vi "Generic LV App Config Save-Retrieve.vi"(8 "error in":errorcluster, 11 "Save/Retrieve":string(combo)="Retrieve") -> (0 "error out":errorcluster, 1 "Path to conf file":path, 2 "Calling VI's Controls":string[](array[string]), 3 "Refs to Calling VI's controls":refnum<vi>[](array[refnum]), 4 "Controls updated":string[](array[string]))   [LabVIEW 2023]
uses:
  <vilib>/Utility/sysdir.llb/System Directory Type.ctl
  <vilib>/Utility/error.llb/Trim Whitespace One-Sided.vi
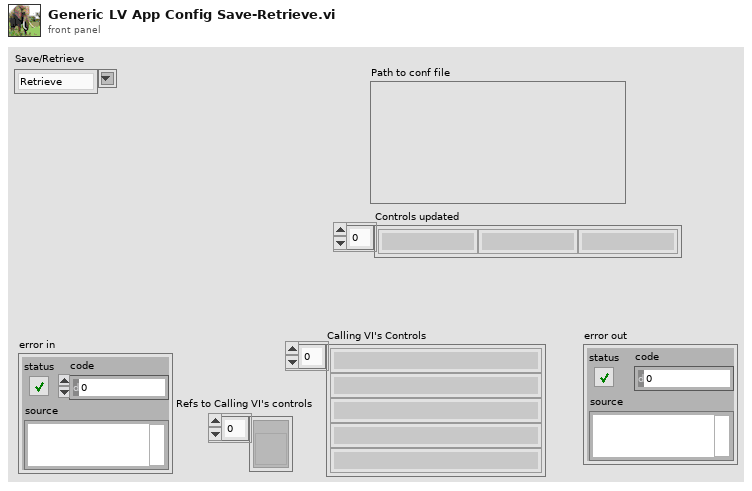
[diagram p1: front panel]
types:
  T1 = enum16{"open", "replace", "create", "open or create", "replace or create", "replace or create with confirmation"}
  T2 = typedef "System Directory Type.ctl" = i32
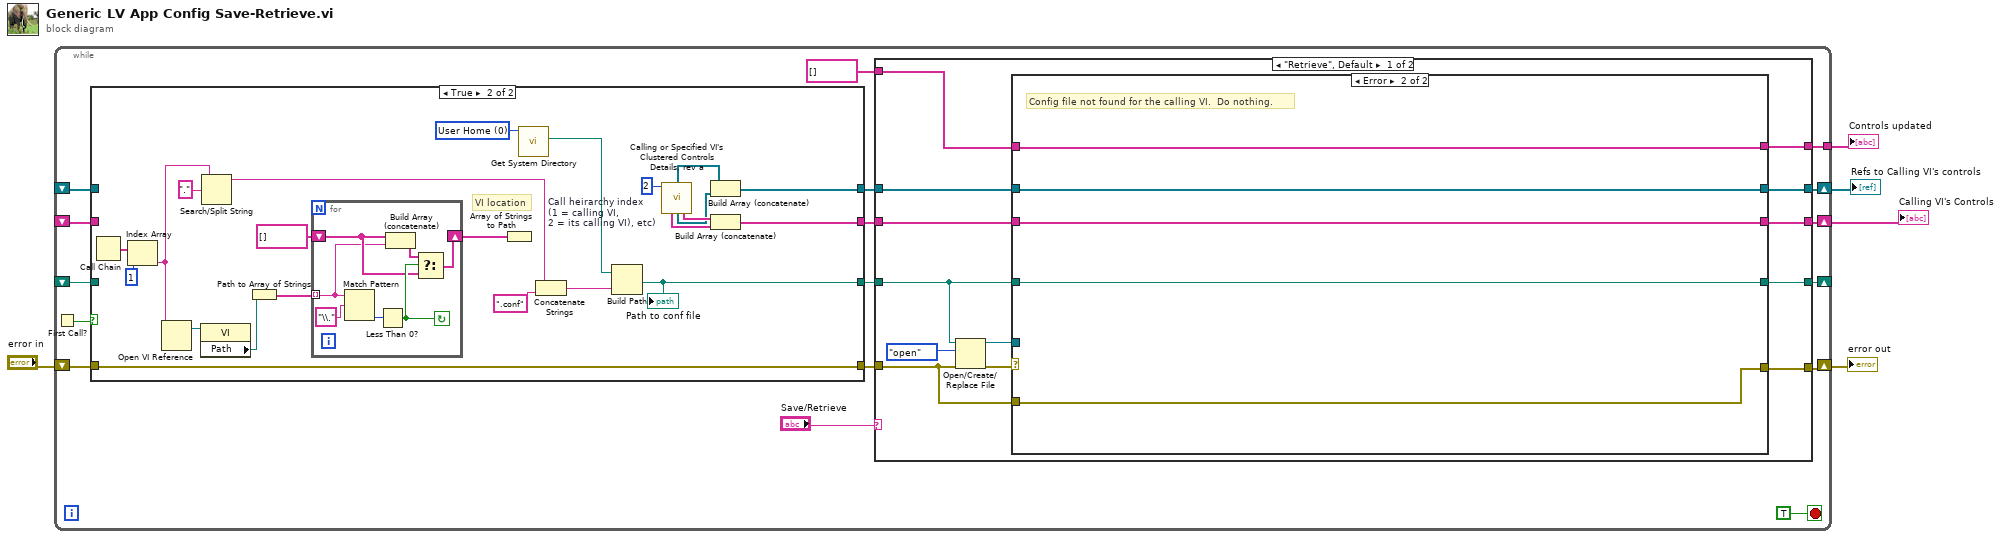
[diagram p0: block diagram]
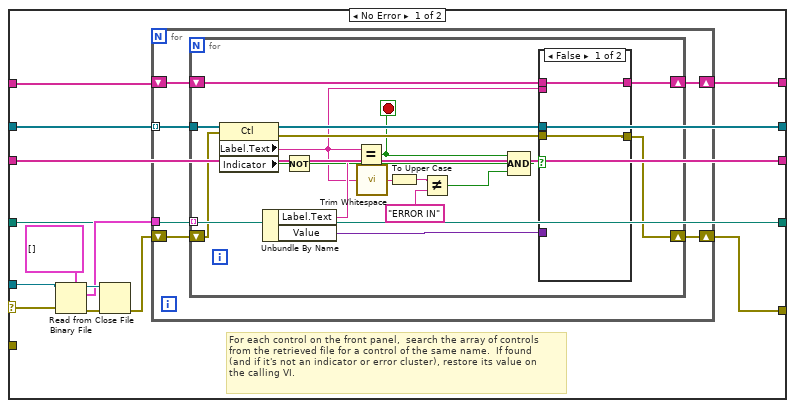
[diagram p3: hidden frame]
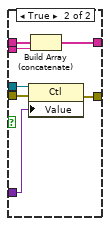
[diagram p4: hidden frame]
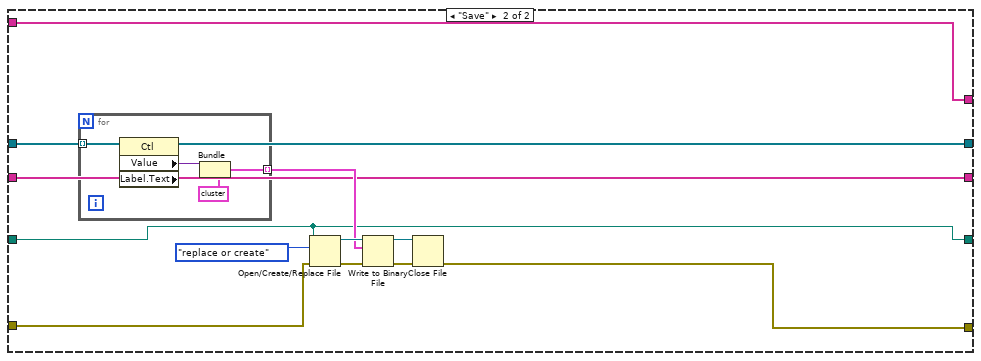
[diagram p5: hidden frame]
diagram:
  n1 = while {
    shift-right: [w15] -> w4
    shift-left: "error in" -> [w18]
    shift-right: [w16] -> w3
    shift-left: _ -> [w12]
    shift-right: [w13] -> w2
    shift-left: _ -> [w11]
    shift-right: [w10] -> _
    shift-left: _ -> [w9]
    tunnel: [w7] -> w1
    stop <- TRUE stop-if-true
    n2 = First Call?() -> (First Call?: T/F=w17:bool)
    n3 = case shown="True" w17 {
      tunnel: [w26 w43] -> w22
      tunnel: [w24 w41] -> w21
      tunnel: [w23 w40] -> w20
      tunnel: w18 -> [w23 w40]
      tunnel: [w25 w39] -> w14
      tunnel: w12 -> [w26 _]
      tunnel: w11 -> [w25 _]
      tunnel: w9 -> [w24 _]
      frame False {
      }
      frame True {
        w28 = T2 0 items=["User Home"=0, "User Desktop"=1, "User Documents"=2, "User Application Data"=3, "User Preferences"=4, "User Temporary"=5, "Public Documents"=6, "Public Application Data"=7, "Public Preferences"=8, "Public Cache"=13, "System Core Libraries"=9, "System Installed Libraries"=10, "Application Files"=11, "Boot Volume Root"=12] ("system directory type")
        w38 = 2  # Call heirarchy index (1 = calling VI,  2 = its calling VI), etc)
        # "VI location"
        n4 = Call Chain() -> (call chain=w49:string[])
        n5 = Index Array(array=w49, index=1) -> (element=w34:string)
        n6 = Open VI Reference(vi path=w34) -> (vi reference=w37:refnum<vi>)  [unwired: 5 in, 1 out]
        n7 = property class="VI"(reference=w37) -> ("Path"=w32:path)  [unwired: 1 in, 2 out]
        n8 = Search/Split String(string=w34, search string/char (-)=".") -> (substring before match=w33:string)  [unwired: 1 in, 2 out]
        n9 = Path to Array of Strings(0:w32) -> (2:w30:string[])  [unwired: 1 out]
        n10 = for {
          tunnel: w30 -> [w50] mode=indexing
          shift-right: [w52] -> w29
          shift-left: string[] [] -> [w51]
          stop <- w54 continue-if-true
          n11 = Match Pattern(string=w50, regular expression="\\.") -> (offset past match=w55:i32)  [unwired: 1 in, 3 out]
          n12 = Less Than 0?(x=w55) -> (x < 0?=w54:bool)
          n13 = Build Array (concatenate)(w51, w50) -> (w53:string[])
          n14 = Select(t=w53, s=w54, f=w51) -> (s? t:f=w52:string[])
        }
        n15 = Array of Strings to Path(0:w29) -> ()  [unwired: 1 in, 1 out]
        n16 = call <vilib>:"Get System Directory.vi"("system directory type"=w28) -> ("system directory"=w27:path)  [unwired: 10 in]
        n17 = Concatenate Strings(w33, ".conf" ("string")) -> (w36:string)
        n18 = Build Path(base path=w27, name or relative path=w36) -> (appended path=w41:path)
        "Path to conf file" <- w41
        n19 = call "Calling or Specified VI's Clustered Controls Details, rev a.vi"("Call heirarchy index\n(1 = calling VI, \n2 = its calling VI), etc)"=w38) -> ("Refs to controls on panel"=w44:refnum<vi>[], "Controls directly on tab panes"=w47:string[], "Refs to controls directly on tab panes"=w45:refnum<vi>[], "Controls on panel"=w46:string[])  [unwired: 5 in, 6 out]
        n20 = Build Array (concatenate)(w44, w45) -> (w43:refnum<vi>[])
        n21 = Build Array (concatenate)(w46, w47) -> (w39:string[])
      }
    }
    n22 = case shown="\"Retrieve\", Default" "Save/Retrieve" {
      tunnel: w22 -> [w66 w124]
      tunnel: w21 -> [w60 w123]
      tunnel: w20 -> [w67 w127]
      tunnel: [w64 w124] -> w16
      tunnel: [w63 w126] -> w15
      tunnel: w14 -> [w62 w125]
      tunnel: [w61 w125] -> w13
      tunnel: [w59 w123] -> w10
      tunnel: [w58 w122] -> w7
      tunnel: string[] [] -> [w57 w122]
      frame "Retrieve", Default {
        n23 = Open/Create/Replace File(file path (use dialog)=w60, error in=w67, operation (0:open)=T1."open") -> (refnum out=w65:refnum<file>, error out=w68:errorcluster)  [unwired: 3 in, 1 out]
        n24 = case shown="Error" w68 {
          selector: w68 -> [w82 _]
          tunnel: w67 -> [_ w121]
          tunnel: [w76 w121] -> w63
          tunnel: w66 -> [w74 w120]
          tunnel: w65 -> [w81 _]
          tunnel: [w74 w120] -> w64
          tunnel: w62 -> [w73 w119]
          tunnel: [w73 w119] -> w61
          tunnel: [w72 w118] -> w59
          tunnel: w60 -> [w72 w118]
          tunnel: [w71 w117] -> w58
          tunnel: w57 -> [w70 w117]
          frame No Error {
            # "For each control on the front panel,  search the array of controls\nfrom the retrieved file for a control of the same name.  If found\n(and if it's not an indicator or error cluster), restore its value on \nthe calling VI."
            n25 = Read from Binary File(5:cluster{"Value":variant, "Label.Text":string}[] [], 8:w82, 11:w81) -> (0:w80:errorcluster, 2:w75:cluster{"Value":variant, "Label.Text":string}[], 3:w79:refnum<file>)  [unwired: 3 in, 1 out]
            n26 = Close File(refnum=w79, error in=w80) -> (error out=w77:errorcluster)  [unwired: 1 out]
            n27 = for {
              tunnel: w74 -> [w88] mode=indexing
              tunnel: w75 -> [w87]
              shift-right: [w85] -> w76
              shift-left: w77 -> [w86]
              shift-right: [w84] -> w71
              shift-left: w70 -> [w83]
              n28 = for {
                tunnel: w88 -> [w107]
                tunnel: w87 -> [w92] mode=indexing
                shift-right: [w101] -> w85
                shift-left: w86 -> [w103]
                shift-right: [w90] -> w84
                shift-left: w83 -> [w89]
                stop <- w99 stop-if-true
                n29 = property class="Ctl"(reference=w107, error in=w103) -> (reference out=w105:refnum<vi>, error out=w102:errorcluster, "Label.Text"=w91:string, "Indicator"=w100:bool)
                n30 = Unbundle By Name(w92) -> ("Label.Text"=w106:string, "Value"=w104:variant)
                n31 = Not(x=w100) -> (.not. x?=w98:bool)
                n32 = Equal?(x=w91, y=w106) -> (x = y?=w99:bool)
                n33 = call <vilib>:"Trim Whitespace.vi"("string"=w91) -> ("trimmed string"=w96:string)  [unwired: 1 in]
                n34 = To Upper Case(1:w96) -> (0:w95:string)
                n35 = Not Equal?(x=w95, y="ERROR IN") -> (x != y?=w93:bool)
                n36 = Compound Arithmetic op=AND(w99, w98, w93) -> (w97:bool)
                n37 = case shown="False" w97 {
                  tunnel: w105 -> [_ w116]
                  tunnel: w104 -> [_ w115]
                  tunnel: w102 -> [w109 w114]
                  tunnel: [w109 w113] -> w101
                  tunnel: w91 -> [_ w112]
                  tunnel: [w108 w111] -> w90
                  tunnel: w89 -> [w108 w110]
                  frame False {
                  }
                  frame True {
                    n38 = property class="Ctl"(reference=w116, error in=w114, "Value"=w115) -> (error out=w113:errorcluster)  [unwired: 1 out]
                    n39 = Build Array (concatenate)(w110, w112) -> (w111:string[])
                  }
                }
              }
            }
          }
          frame Error {
            # "Config file not found for the calling VI.  Do nothing."
          }
        }
      }
      frame "Save" {
        n40 = for {
          tunnel: w124 -> [w138] mode=indexing
          tunnel: [w134] -> w130 mode=indexing
          n41 = property class="Ctl"(reference=w138) -> ("Value"=w137:variant, "Label.Text"=w136:string)  [unwired: 1 in, 2 out]
          n42 = Bundle(cluster=cluster{"Value":variant, "Label.Text":string} {"Value"=variant, "Label.Text"=""}, "Value"=w137, "Label.Text"=w136) -> (w134:cluster{"Value":variant, "Label.Text":string})
        }
        n43 = Open/Create/Replace File(file path (use dialog)=w123, error in=w127, operation (0:open)=T1."replace or create") -> (refnum out=w132:refnum<file>, error out=w131:errorcluster)  [unwired: 3 in, 1 out]
        n44 = Write to Binary File(file (use dialog)=w132, data=w130, error in=w131) -> (refnum out=w129:refnum<file>, error out=w128:errorcluster)  [unwired: 3 in, 1 out]
        n45 = Close File(refnum=w129, error in=w128) -> (error out=w126:errorcluster)  [unwired: 1 out]
      }
    }
  }
  "error out" <- w4
  "Refs to Calling VI's controls" <- w3
  "Calling VI's Controls" <- w2
  "Controls updated" <- w1
